vi "Resolve Seconds Wait.vi"(8 "error in (no error)":errorcluster, 11 "Settings in":T1 {"Channel Refnum" format="%.0x"; "Linked Channels"."Channel Refnum" format="%.0x"}) -> (0 "error out":errorcluster, 1 "Wait value (sec)":dbl, 2 "Channel Path":string, 3 "Settings out":T1 {"Channel Refnum" format="%.0x"; "Linked Channels"."Channel Refnum" format="%.0x"})   [LabVIEW 2018, in "Instrument Addon Scripting API.lvlib"]
uses:
  Instrument Addon Scripting API.lvlib
  TypeDefs/Wait Response Settings.ctl
  TypeDefs/Linked Channel.ctl
  <vilib>/NI Veristand/Custom Device API/Custom Device Item Ref.ctl
  NationalInstruments.VeriStand.SystemStorage
  Addon/Addon System Explorer/Instrument Addon System Explorer.lvlib
  <vilib>/NI Veristand/Custom Device API/Custom Device API.lvlib
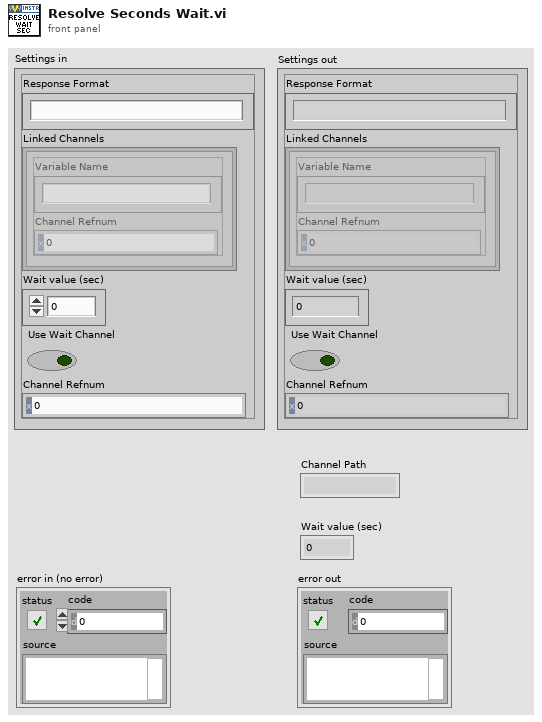
[diagram p1: front panel]
types:
  T1 = typedef "Instrument Addon Scripting API.lvlib/Wait Response Settings.ctl" = cluster{"Response Format":string, "Linked Channels":T2[], "Wait value (sec)":dbl, "Use Wait Channel":bool, "Channel Refnum":T3}
  T2 = typedef "Instrument Addon Scripting API.lvlib/Linked Channel.ctl" = cluster{"Variable Name":string, "Channel Refnum":T3}
  T3 = typedef "Custom Device API.lvlib/Custom Device Item Ref.ctl" = u64
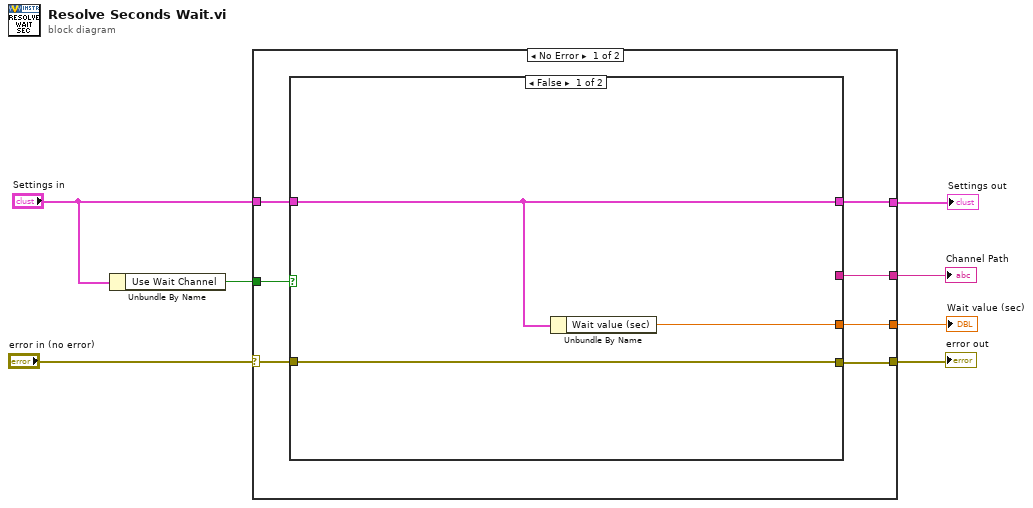
[diagram p0: block diagram]
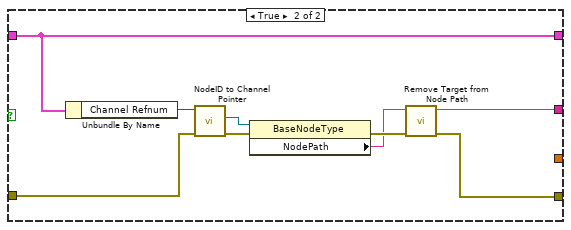
[diagram p2: hidden frame]
diagram:
  n1 = Unbundle By Name("Settings in") -> ("Use Wait Channel"=w5:bool)
  n2 = case shown="No Error" "error in (no error)" {
    selector: "error in (no error)" -> [w12 w27]
    tunnel: "Settings in" -> [w13 w28]
    tunnel: w5 -> [w14 _]
    tunnel: [w11 w27] -> w7
    tunnel: [w10 w28] -> w2
    tunnel: [w9 _] -> w6
    tunnel: [w8 _] -> w1
    frame No Error {
      n3 = case shown="False" w14 {
        tunnel: w13 -> [w17 w19]
        tunnel: w12 -> [w15 w23]
        tunnel: [w15 w20] -> w11
        tunnel: [w17 w19] -> w10
        tunnel: [_ w18] -> w9
        tunnel: [w16 _] -> w8
        frame False {
          n4 = Unbundle By Name(w17) -> ("Wait value (sec)"=w16:dbl)
        }
        frame True {
          n5 = Unbundle By Name(w19) -> ("Channel Refnum"=w26:T3)
          n6 = call "NodeID to Channel Pointer.vi"("error in (no error)"=w23, "nodeID in"=w26) -> ("error out"=w22:errorcluster, "BaseNodeType out"=w21:refnum<k24>)  [unwired: 7 in, 1 out]
          n7 = property class="BaseNodeType"(reference=w21, error in=w22) -> (error out=w25:errorcluster, "NodePath"=w24:string)  [unwired: 1 out]
          n8 = call "Remove Target from Node Path.vi"("error in (no error)"=w25, "NodePath"=w24) -> ("error out"=w20:errorcluster, "PathArrayToString"=w18:string)  [unwired: 8 in]
        }
      }
    }
    frame Error {
    }
  }
  "error out" <- w7
  "Channel Path" <- w6
  "Settings out" <- w2
  "Wait value (sec)" <- w1
